vi "Globals.vi"() -> ()   [LabVIEW 2011, in "Switch-DMM Custom Device.lvlib"]
uses:
  Switch-DMM Custom Device.lvlib
panel:
  in  "Current Samples":string="Current Samples"
  in  "Auto-Read":string="Auto-Read"
  in  "Trigger Channel":string="Trigger Channel"
  in  "Mode Channel":string="Mode Channel"
  in  "Current Limit":string="Current Limit"
  in  "Current Read Rate":string="Current Read Rate"
  in  "DMM-Switch Trig":string="DMM-Switch Trig"
  in  "Switch-DMM Trig":string="Switch-DMM Trig"
  in  "Current Channel":string="Current Channel"
  in  "DMM Device":string="DMM Device"
  in  "Switch Device":string="Switch Device"
  in  "Voltage Section":string="Voltage Section"
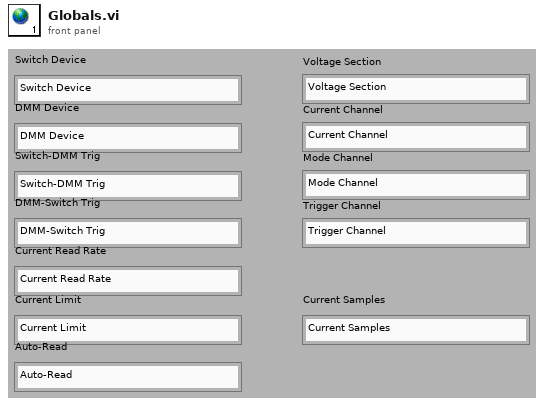
[diagram p1: front panel]
diagram:
